vi "Find Attribute.vi"() -> ()   [LabVIEW 2023]
panel:
  in  "Directory Path":path=path "E:/Dev/ni-central/src/rfmx"
  in  "Attribute Hex ID":string="A040DE"
  out "XML File Path/s":path[](array[path])
  out "text":string
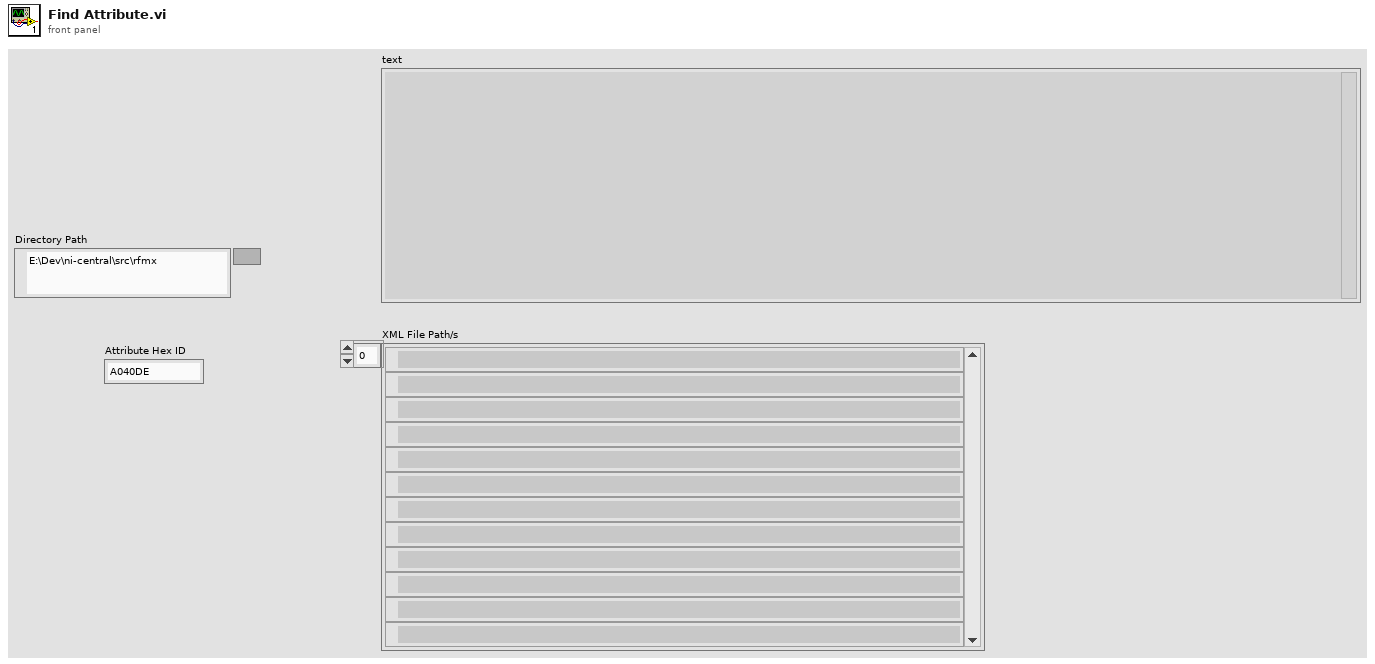
[diagram p1: front panel]
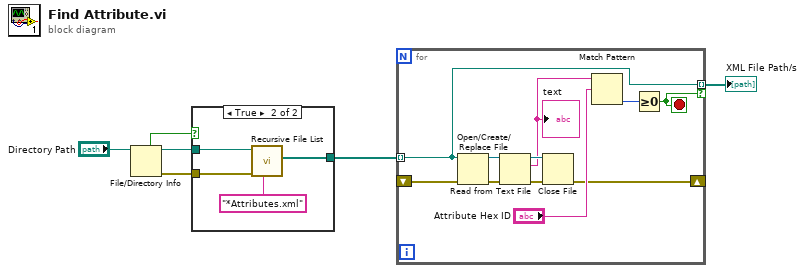
[diagram p0: block diagram]
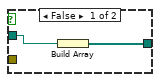
[diagram p2: hidden frame]
diagram:
  n1 = File/Directory Info(path="Directory Path") -> (path out=w3:path, directory=w1:bool, error out=w2:errorcluster)  [unwired: 1 in, 4 out]
  n2 = case shown="True" w1 {
    tunnel: [w7 w11] -> w6
    tunnel: w3 -> [w8 w10]
    tunnel: w2 -> [_ w9]
    frame False {
      n3 = Build Array(w8) -> (w7:path[])
    }
    frame True {
      n4 = call <vilib>:"Recursive File List.vi"("pattern"="*Attributes.xml", "error in (no error)"=w9, "Folder Path"=w10) -> ("All Files in Dir"=w11:path[])  [unwired: 4 in, 4 out]
    }
  }
  n5 = for {
    tunnel: w6 -> [w16] mode=indexing
    tunnel: [w16] -> w5 mode=indexing if=w15
    shift-right: [w13] -> _
    shift-left: _ -> [w14]
    stop <- w15 stop-if-true
    n6 = Open/Create/Replace File(file path (use dialog)=w16, error in=w14) -> (refnum out=w23:refnum<file>, error out=w22:errorcluster)  [unwired: 4 in, 1 out]
    n7 = Read from Text File(file (use dialog)=w23, error in=w22) -> (refnum out=w21:refnum<file>, text=w19:string, error out=w20:errorcluster)  [unwired: 2 in, 1 out]
    "text" <- w19
    n8 = Close File(refnum=w21, error in=w20) -> (error out=w13:errorcluster)  [unwired: 1 out]
    n9 = Match Pattern(string=w19, regular expression="Attribute Hex ID") -> (offset past match=w17:i32)  [unwired: 1 in, 3 out]
    n10 = Greater Or Equal To 0?(x=w17) -> (x >= 0?=w15:bool)
  }
  "XML File Path/s" <- w5
